vi "Add User.vi"(0 "User Manager Model in":refnum<class "User Manager Model.lvclass">, 5 "User Info":T2, 7 "User Level":T1, 11 "error in (no error)":errorcluster) -> (4 "User Manager Model out":refnum<class "User Manager Model.lvclass">, 15 "error out":errorcluster)   [LabVIEW 2017, in "User Manager Model.lvlib" / "User Manager Model.lvclass"]
uses:
  User Manager Model.lvclass
  C:/Program Files/National Instruments/LabVIEW 2017/vi.lib/ActorFramework/Actor/Actor.lvclass
  Type Definitions/Credentials.ctl
  Type Definitions/User Levels.ctl
  User Manager Model Messages/Get All Users Msg/Get All Users Msg.lvclass
  C:/Program Files/National Instruments/LabVIEW 2017/vi.lib/ActorFramework/Message/Message.lvclass
  User Manager Model Messages/Save Msg/Save Msg.lvclass
  <vilib>/ActorFramework/Actor/Actor.lvclass/Actor.ctl
  <vilib>/ActorFramework/Message Enqueuer/Message Enqueuer.lvclass/Message Enqueuer.ctl
  User Manager Model.lvclass/User Manager Model.ctl
  <vilib>/ActorFramework/Message Enqueuer/Init from Existing Queue.vi
  <vilib>/ActorFramework/Message Priority Queue/Priority Enqueue.vi
  <vilib>/ActorFramework/Message Enqueuer/Message Enqueuer.lvclass
  <vilib>/gpm_packages/@cs/user-manager/Source/User Configuration Manager Ref/By Ref.lvlib
  <vilib>/ActorFramework/Actor/Actor.lvclass
  Type Definitions/User Manager Application Types.lvlib
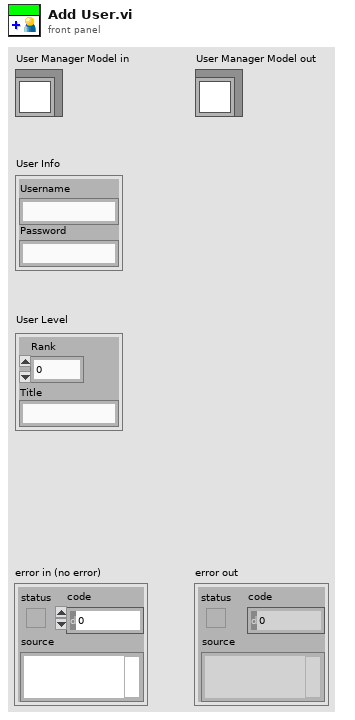
[diagram p1: front panel]
types:
  T1 = typedef "User Manager Application Types.lvlib/User Levels.ctl" = cluster{"Rank":i32, "Title":string}
  T2 = typedef "User Manager Application Types.lvlib/Credentials.ctl" = cluster{"Username":string, "Password":string}
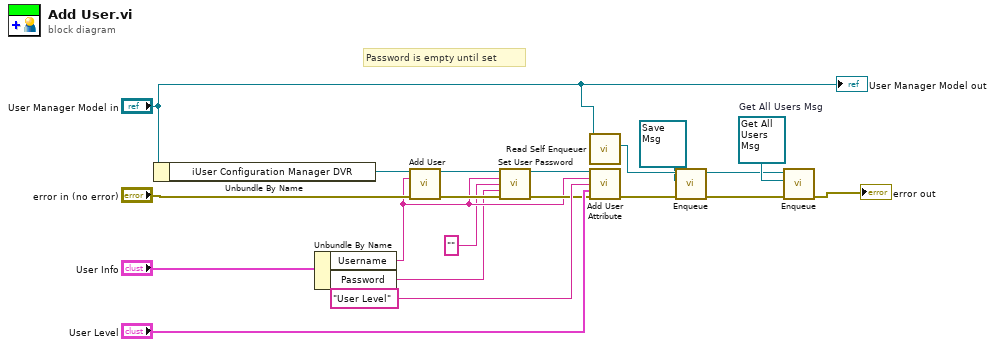
[diagram p0: block diagram]
diagram:
  w9 = refnum<class "Get All Users Msg.lvclass"> refnum  # Get All Users Msg
  # "Password is empty until set"
  n1 = Unbundle By Name("User Manager Model in") -> ("iUser Configuration Manager DVR"=w20:refnum<data-value>)
  n2 = Unbundle By Name("User Info") -> ("Username"=w3:string, "Password"=w2:string)
  n3 = call <vilib>:"Add User.vi"("iUser Configuration Manager DVR"=w20, "Username"=w3, "error in"="error in (no error)") -> ("dup iUser Configuration Manager DVR"=w18:refnum<data-value>, "error out"=w14:errorcluster)  [unwired: 10 in, 1 out]
  n4 = call <vilib>:"Set User Password.vi"("iUser Configuration Manager DVR"=w18, "Username"=w3, "Current Password"="", "New Password"=w2, "error in"=w14) -> ("dup iUser Configuration Manager DVR"=w17:refnum<data-value>, "error out"=w13:errorcluster)  [unwired: 8 in, 1 out]
  n5 = call <vilib>:"Read Self Enqueuer.vi"("Actor"="User Manager Model in") -> ("Self Enqueuer"=w8:refnum<class "Message Enqueuer.lvclass">)  [unwired: 10 in]
  n6 = call <vilib>:"Add User Attribute.vi"("iUser Configuration Manager DVR"=w17, "Username"=w3, "Attribute Name"="User Level", "Attribute Value"="User Level", "error in"=w13) -> ("error out"=w5:errorcluster)  [unwired: 8 in, 2 out]
  n7 = call <vilib>:"Enqueue.vi"("error in (no error)"=w5, "Message"=refnum<class "Save Msg.lvclass"> refnum ("User Manager Model.lvlib:Save Msg.lvclass"), "Message Enqueuer in"=w8) -> ("error out"=w4:errorcluster, "Message Enqueuer out"=w7:refnum<class "Message Enqueuer.lvclass">)  [unwired: 7 in]
  n8 = call <vilib>:"Enqueue.vi"("error in (no error)"=w4, "Message"=w9, "Message Enqueuer in"=w7) -> ("error out"=→"error out":errorcluster)  [unwired: 7 in, 1 out]
  "User Manager Model out" <- "User Manager Model in"
